vi "host.vi"() -> ()   [LabVIEW 2020]
uses:
  <vilib>/FPGAPlugInAG/cRIO-9035/niLvFpga_Open_cRIO-9035.vi
  <vilib>/rvi/interface/common/dynamic/niFpgaDynamicAddResources.vi
  <vilib>/Utility/error.llb/Error Cluster From Error Code.vi
  <vilib>/rvi/errors/niLvFpgaAdjustHostInterfaceError.vi
  <vilib>/FPGAPlugInAG/Dynamic/niLvFpga_Run_Dynamic.vi
  <vilib>/FPGAPlugInAG/Dynamic/niLvFpga_Reset_Dynamic.vi
  <vilib>/FPGAPlugInAG/Dynamic/niLvFpga_Close_Dynamic.vi
  <vilib>/rvi/interface/nirviOpenFPGA/nirviOpenFPGA.xnode
  FPGA Bitfiles/fftfpgaapplicati_FPGATarget_FFT2_lowKbXhkvqo.lvbitx
  FFT.vi
  <vilib>/rvi/interface/nirviMethod/nirviMethod.xnode
  <vilib>/rvi/interface/nirviCloseFPGA/nirviCloseFPGA.xnode
  <vilib>/rvi/errors/niLvFpgaMergeErrorWithErrorCode.vi
  <vilib>/FPGAPlugInAG/Dynamic/niLvFpga_ReadFifo_Dynamic.vi
  <vilib>/Analysis/NI_AALPro.lvlib
  <vilib>/FPGAPlugInAG/Dynamic/niLvFpga_StartFifo_Dynamic.vi
  <vilib>/FPGAPlugInAG/Dynamic/niLvFpga_WriteFifo_Dynamic.vi
panel:
  out "signal_target_to_host_fixed size(s)":i32
  out "Elements Remaining":u32
  out "Array":fxp<+/-,24,7>[](array[numeric])
  out "signal target to host":dbl[][](graph)
  out "data collection time":u32[](array[numeric])
  out "FFT time":u32[](array[numeric])
  out "signal_target_to_host_fixed":fxp<+/-,24,7>[](array[numeric])
  out "real array size":i32
  out "imaginaryDBL array size":i32
  out "real Fixed":fxp<+/-,32,21>[](array[numeric])
  out "imaginary Fixed":fxp<+/-,32,21>[](array[numeric])
  out "detrend acc":dbl[](graph)
  out "acc":dbl[](graph)
  out "samples":i32
  out "Waveform Graph":dbl[][](graph)
  out "input signal":T1(graph)
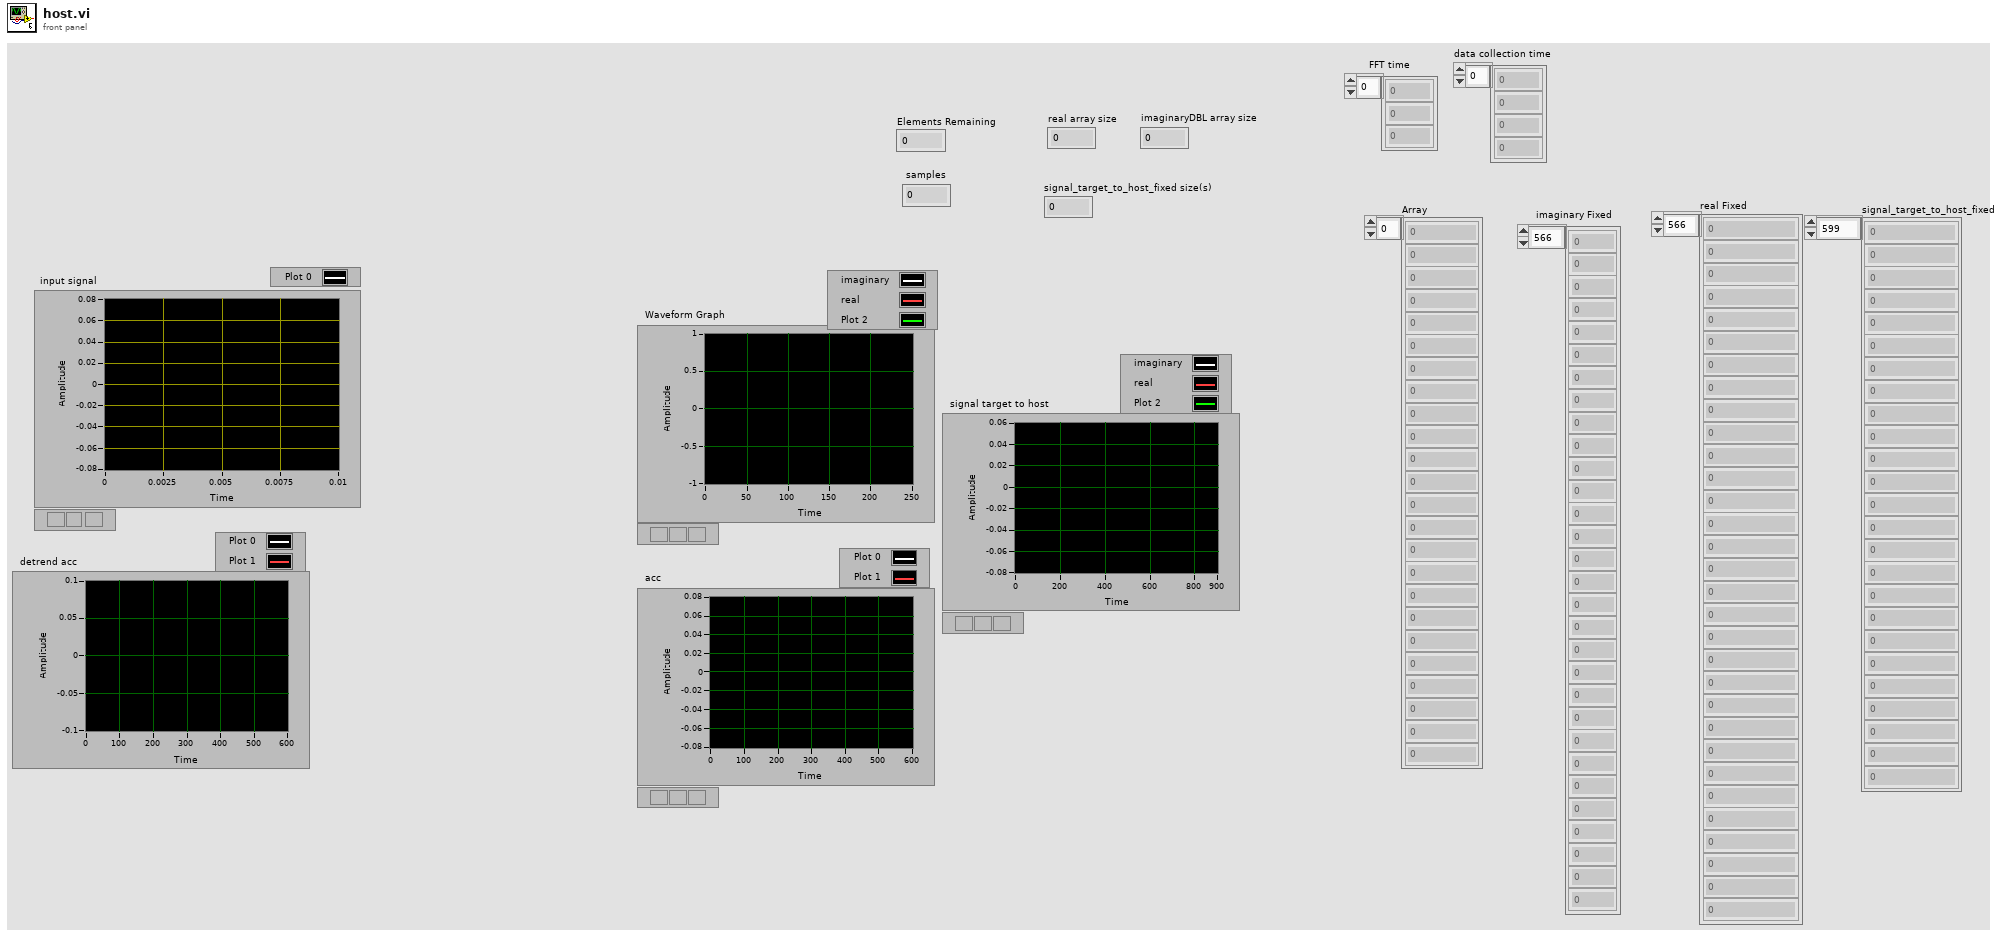
[diagram p1: front panel]
types:
  T1 = cluster{"array type (2D Dbl)":dbl[], "array type (2D Dbl)":dbl[]}
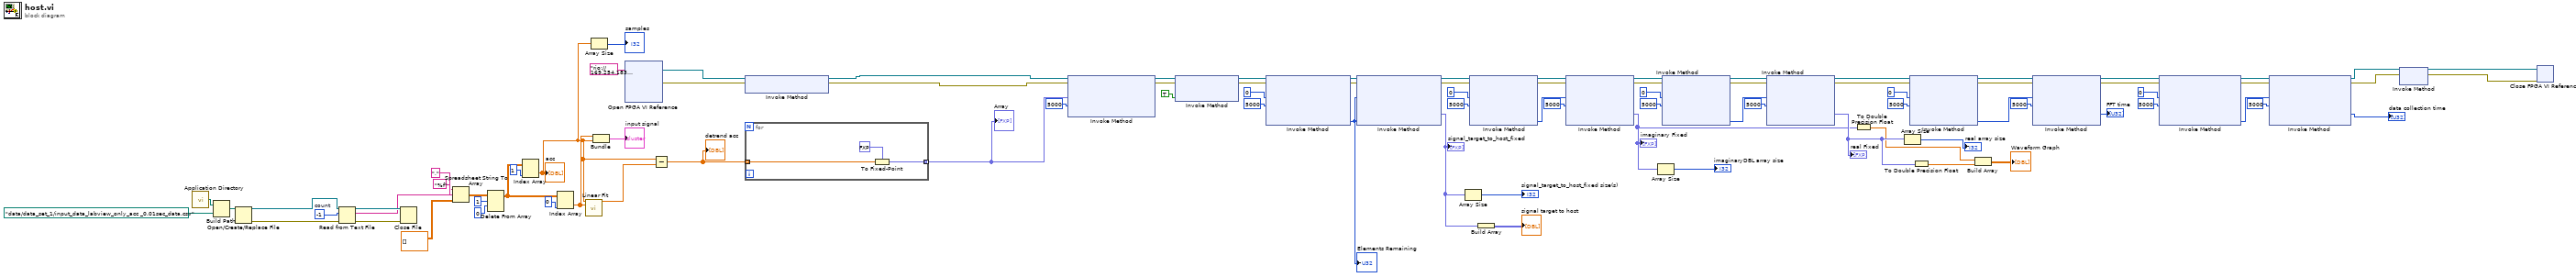
[diagram p0: block diagram]
diagram:
  w80 = -1  # count
  n1 = call <vilib>:"Application Directory.vi"() -> ("Application Directory"=w84:path)
  n2 = Build Path(base path=w84, name or relative path=path "data/data_set_1/input_data_labview_only_acc _0.01sec_data.csv" ("default name")) -> (appended path=w83:path)
  n3 = Open/Create/Replace File(file path (use dialog)=w83) -> (refnum out=w88:refnum<file>, error out=w89:errorcluster)  [unwired: 5 in, 1 out]
  n4 = Read from Text File(file (use dialog)=w88, count=w80, error in=w89) -> (refnum out=w87:refnum<file>, text=w85:string, error out=w86:errorcluster)  [unwired: 1 in, 1 out]
  n5 = Close File(refnum=w87, error in=w86) -> ()  [unwired: 2 out]
  n6 = Spreadsheet String To Array(delimiter (Tab)=",", format string="%f", spreadsheet string=w85, array type (2D Dbl)=dbl[][] []) -> (array=w77:dbl[][])
  n7 = Delete From Array(array=w77, length=1, index (row)=0) -> (array with subset deleted=w72:dbl[][])  [unwired: 1 in, 1 out]
  n8 = Index Array(array=w72, index (col)=1 ("disabled index (col)")) -> (element=w43:dbl[])  [unwired: 1 in]
  "acc" <- w43
  n9 = Index Array(array=w72, index (col)=0 ("disabled index (col)")) -> (element=w46:dbl[])  [unwired: 1 in]
  n10 = call <vilib>:"Linear Fit.vi"("Y"=w43, "X"=w46) -> ("Best Linear Fit"=w44:dbl[])  [unwired: 9 in, 4 out]
  n11 = Array Size(array=w43) -> (size(s)=→"samples":i32)
  n12 = Bundle("array type (2D Dbl)"=w46, "array type (2D Dbl)"=w43) -> (→"input signal":T1)  [unwired: 1 in]
  n13 = xnode "Open FPGA VI Reference"("resource name"=tag "rio://169.254.183.73/RIO0") -> ("FPGA VI Reference Out"=w8:refnum<k20>, "error out"=w7:errorcluster)  [unwired: 1 in]
  n14 = Subtract(x=w43, y=w44) -> (x-y=w45:dbl[])
  "detrend acc" <- w45
  n15 = xnode "Invoke Method"("FPGA VI Reference In"=w8, "error in"=w7) -> ("FPGA VI Reference Out"=w2:refnum<k20>, "error out"=w1:errorcluster)
  n16 = for {
    tunnel: [w91] -> w31 mode=indexing
    tunnel: w45 -> [w90] mode=indexing
    n17 = To Fixed-Point(fixed-point type=fxp<+/-,24,7> 0.0 ("f"), number=w90) -> (fixed-point=w91:fxp<+/-,24,7>)
  }
  "Array" <- w31
  n18 = xnode "Invoke Method"("FPGA VI Reference In"=w2, "error in"=w1, "Data"=w31, "Timeout (ms)"=5000) -> ("FPGA VI Reference Out"=w69:refnum<k20>, "error out"=w68:errorcluster)  [unwired: 1 out]
  n19 = xnode "Invoke Method"("FPGA VI Reference In"=w69, "error in"=w68, "Wait Until Done (F)"=TRUE) -> ("FPGA VI Reference Out"=w32:refnum<k20>, "error out"=w33:errorcluster)
  n20 = xnode "Invoke Method"("FPGA VI Reference In"=w32, "error in"=w33, "Number of Elements"=u32 0, "Timeout (ms)"=5000) -> ("FPGA VI Reference Out"=w36:refnum<k20>, "error out"=w35:errorcluster, "Elements Remaining"=w34:u32)  [unwired: 1 out]
  "Elements Remaining" <- w34
  n21 = xnode "Invoke Method"("FPGA VI Reference In"=w36, "error in"=w35, "Number of Elements"=w34) -> ("FPGA VI Reference Out"=w30:refnum<k20>, "error out"=w29:errorcluster, "Data"=w10:fxp<+/-,24,7>[])  [unwired: 1 in, 1 out]
  "signal_target_to_host_fixed" <- w10
  n22 = Array Size(array=w10) -> (size(s)=→"signal_target_to_host_fixed size(s)":i32)
  n23 = xnode "Invoke Method"("FPGA VI Reference In"=w30, "error in"=w29, "Number of Elements"=u32 0, "Timeout (ms)"=5000) -> ("FPGA VI Reference Out"=w67:refnum<k20>, "error out"=w66:errorcluster, "Elements Remaining"=w60:u32)  [unwired: 1 out]
  n24 = Build Array(w10) -> (→"signal target to host":fxp<+/-,24,7>[][])
  n25 = xnode "Invoke Method"("FPGA VI Reference In"=w67, "error in"=w66, "Number of Elements"=w60, "Timeout (ms)"=5000) -> ("FPGA VI Reference Out"=w63:refnum<k20>, "error out"=w62:errorcluster, "Data"=w39:fxp<+/-,28,11>[])  [unwired: 1 out]
  "imaginary Fixed" <- w39
  n26 = Array Size(array=w39) -> (size(s)=→"imaginaryDBL array size":i32)
  n27 = xnode "Invoke Method"("FPGA VI Reference In"=w63, "error in"=w62, "Number of Elements"=u32 0, "Timeout (ms)"=5000) -> ("FPGA VI Reference Out"=w65:refnum<k20>, "error out"=w64:errorcluster, "Elements Remaining"=w58:u32)  [unwired: 1 out]
  n28 = xnode "Invoke Method"("FPGA VI Reference In"=w65, "error in"=w64, "Number of Elements"=w58, "Timeout (ms)"=5000) -> ("FPGA VI Reference Out"=w55:refnum<k20>, "error out"=w54:errorcluster, "Data"=w40:fxp<+/-,28,11>[])  [unwired: 1 out]
  "real Fixed" <- w40
  n29 = To Double Precision Float(number=w39) -> (double precision float=w37:dbl[])
  n30 = Array Size(array=w40) -> (size(s)=→"real array size":i32)
  n31 = xnode "Invoke Method"("FPGA VI Reference In"=w55, "error in"=w54, "Number of Elements"=u32 0, "Timeout (ms)"=5000) -> ("FPGA VI Reference Out"=w26:refnum<k20>, "error out"=w25:errorcluster, "Elements Remaining"=w24:u32)  [unwired: 1 out]
  n32 = To Double Precision Float(number=w40) -> (double precision float=w38:dbl[])
  n33 = Build Array(w37, w38) -> (→"Waveform Graph":dbl[][])
  n34 = xnode "Invoke Method"("FPGA VI Reference In"=w26, "error in"=w25, "Number of Elements"=w24, "Timeout (ms)"=5000) -> ("FPGA VI Reference Out"=w22:refnum<k20>, "error out"=w21:errorcluster, "Data"=→"FFT time":u32[])  [unwired: 1 out]
  n35 = xnode "Invoke Method"("FPGA VI Reference In"=w22, "error in"=w21, "Number of Elements"=u32 0, "Timeout (ms)"=5000) -> ("FPGA VI Reference Out"=w20:refnum<k20>, "error out"=w19:errorcluster, "Elements Remaining"=w18:u32)  [unwired: 1 out]
  n36 = xnode "Invoke Method"("FPGA VI Reference In"=w20, "error in"=w19, "Number of Elements"=w18, "Timeout (ms)"=5000) -> ("FPGA VI Reference Out"=w6:refnum<k20>, "error out"=w5:errorcluster, "Data"=→"data collection time":u32[])  [unwired: 1 out]
  n37 = xnode "Invoke Method"("FPGA VI Reference In"=w6, "error in"=w5) -> ("FPGA VI Reference Out"=w4:refnum<k20>, "error out"=w3:errorcluster)
  n38 = xnode "Close FPGA VI Reference"("FPGA VI Reference In"=w4, "error in"=w3) -> ()  [unwired: 1 out]
